vi "Close.vi"(8 "error in (no error)":errorcluster, 11 "VISA Tegam4040":refnum<visa-resource-name>) -> (0 "error out":errorcluster)   [LabVIEW 2010]
doc: "Closes a device session or event object specified by VISA resource name. For each VISA session that you open, you should close the session when you are finished with it. This function accepts all available classes."
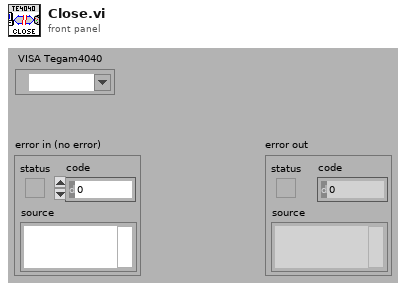
[diagram p1: front panel]
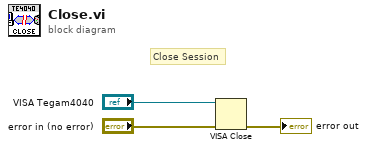
[diagram p0: block diagram]
diagram:
  # "Close Session"
  n1 = VISA Close(VISA resource name="VISA Tegam4040", error in (no error)="error in (no error)") -> (error out=→"error out":errorcluster)
